vi "Get Generic Property.vi"   [LabVIEW 2020, in "SLSC.lvlib"]
doc: "Gets the value of the specified device property for one or more resources. This is flexible for devices, NVMEM, physical channels, and so on, but requires that you know the exact string of the resource. You can use an array instance of this VI to get a scalar property from multiple devices with a single call to the VI."
uses:
  <vilib>/SLSC/SLSC.lvlib
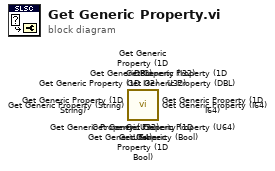
[diagram p0: block diagram]
diagram:
  n1 = call <vilib>:"Get Generic Property (1D U64).vi"() -> ()  [unwired: 13 in, 3 out]
  n2 = call <vilib>:"Get Generic Property (1D U32).vi"() -> ()  [unwired: 13 in, 3 out]
  n3 = call <vilib>:"Get Generic Property (1D String).vi"() -> ()  [unwired: 13 in, 3 out]
  n4 = call <vilib>:"Get Generic Property (1D I64).vi"() -> ()  [unwired: 13 in, 3 out]
  n5 = call <vilib>:"Get Generic Property (1D I32).vi"() -> ()  [unwired: 13 in, 3 out]
  n6 = call <vilib>:"Get Generic Property (1D DBL).vi"() -> ()  [unwired: 13 in, 3 out]
  n7 = call <vilib>:"Get Generic Property (1D Bool).vi"() -> ()  [unwired: 13 in, 3 out]
  n8 = call <vilib>:"Get Generic Property (U64).vi"() -> ()  [unwired: 13 in, 3 out]
  n9 = call <vilib>:"Get Generic Property (U32).vi"() -> ()  [unwired: 13 in, 3 out]
  n10 = call <vilib>:"Get Generic Property (String).vi"() -> ()  [unwired: 13 in, 3 out]
  n11 = call <vilib>:"Get Generic Property (I64).vi"() -> ()  [unwired: 13 in, 3 out]
  n12 = call <vilib>:"Get Generic Property (I32).vi"() -> ()  [unwired: 13 in, 3 out]
  n13 = call <vilib>:"Get Generic Property (DBL).vi"() -> ()  [unwired: 13 in, 3 out]
  n14 = call <vilib>:"Get Generic Property (Bool).vi"() -> ()  [unwired: 13 in, 3 out]
